vi "Init DAQs.vi"(8 "error in (no error)":errorcluster, 11 "Timing":T1={"Sampling Rate (Hz)"=1000.0, "Samples to Read"=100, "Sampling Mode"=2} {"Sampling Mode" items=["Finite Samples", "Continuous Samples", "Hardware Timed Single Point"]; "Sampling Rate (Hz)" format="%0.2f"}) -> (0 "error out":errorcluster, 2 "Channel Array":refnum<k21>[](array[refnum]))   [LabVIEW 2017]
uses:
  Controls/Timing Controls.ctl
  <vilib>/DAQmx/create/channels.llb/DAQmx Create Channel (AI-Voltage-Basic).vi
  <vilib>/DAQmx/configure/timing.llb/DAQmx Timing (Sample Clock).vi
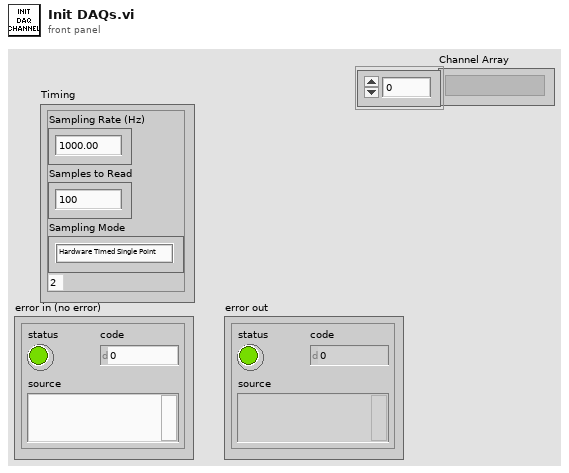
[diagram p1: front panel]
types:
  T1 = typedef "Timing Controls.ctl" = cluster{"Sampling Rate (Hz)":dbl, "Samples to Read":i32, "Sampling Mode":i32}
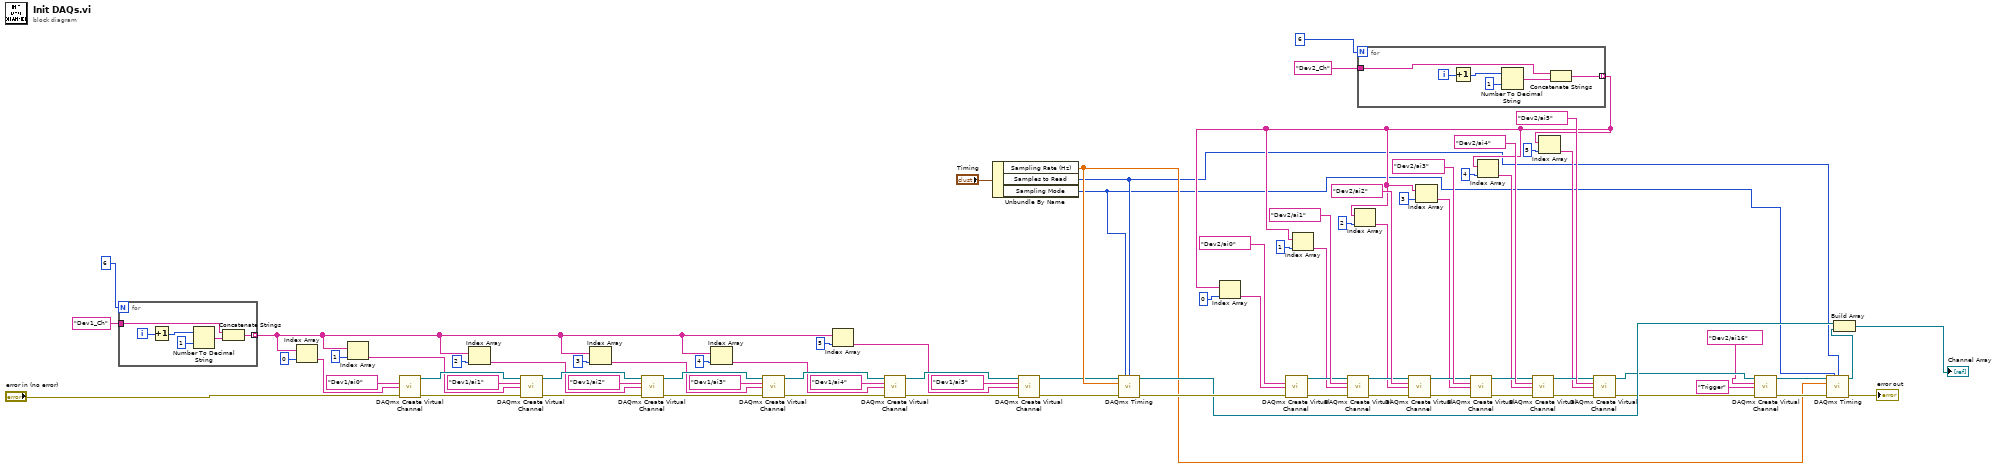
[diagram p0: block diagram]
diagram:
  n1 = for {
    N: 6 -> [_]
    tunnel: "Dev1_Ch" ("name to assign") -> [w82]
    tunnel: [w81] -> w6 mode=indexing
    i -> [w86]
    n2 = Increment(x=w86) -> (x+1=w84:i32)
    n3 = Number To Decimal String(number=w84, width (-)=i16 1) -> (decimal integer string=w83:string)
    n4 = Concatenate Strings(w82, w83) -> (w81:string)
  }
  n5 = Index Array(array=w6, index=0) -> (element=w12:string)
  n6 = Index Array(array=w6, index=1) -> (element=w5:string)
  n7 = call-poly <vilib>:"DAQmx Create Virtual Channel.vi"("physical channels"=tag "Dev1/ai0", "name to assign"=w12, "error in"="error in (no error)") -> ("task out"=w33:refnum<k21>, "error out"=w29:errorcluster)  [unwired: 11 in]
  n8 = Index Array(array=w6, index=2) -> (element=w4:string)
  n9 = call-poly <vilib>:"DAQmx Create Virtual Channel.vi"("task in"=w33, "physical channels"=tag "Dev1/ai1", "name to assign"=w5, "error in"=w29) -> ("task out"=w31:refnum<k21>, "error out"=w27:errorcluster)  [unwired: 10 in]
  n10 = Index Array(array=w6, index=3) -> (element=w3:string)
  n11 = call-poly <vilib>:"DAQmx Create Virtual Channel.vi"("task in"=w31, "physical channels"=tag "Dev1/ai2", "name to assign"=w4, "error in"=w27) -> ("task out"=w30:refnum<k21>, "error out"=w25:errorcluster)  [unwired: 10 in]
  n12 = Index Array(array=w6, index=4) -> (element=w2:string)
  n13 = call-poly <vilib>:"DAQmx Create Virtual Channel.vi"("task in"=w30, "physical channels"=tag "Dev1/ai3", "name to assign"=w3, "error in"=w25) -> ("task out"=w22:refnum<k21>, "error out"=w23:errorcluster)  [unwired: 10 in]
  n14 = Index Array(array=w6, index=5) -> (element=w1:string)
  n15 = call-poly <vilib>:"DAQmx Create Virtual Channel.vi"("task in"=w22, "physical channels"=tag "Dev1/ai4", "name to assign"=w2, "error in"=w23) -> ("task out"=w19:refnum<k21>, "error out"=w18:errorcluster)  [unwired: 10 in]
  n16 = Unbundle By Name("Timing") -> ("Sampling Rate (Hz)"=w37:dbl, "Samples to Read"=w36:i32, "Sampling Mode"=w35:i32)
  n17 = call-poly <vilib>:"DAQmx Create Virtual Channel.vi"("task in"=w19, "physical channels"=tag "Dev1/ai5", "name to assign"=w1, "error in"=w18) -> ("task out"=w17:refnum<k21>, "error out"=w16:errorcluster)  [unwired: 10 in]
  n18 = call-poly <vilib>:"DAQmx Timing.vi"("task/channels in"=w17, "sample mode"=w35, "samples per channel"=w36, "rate"=w37, "error in"=w16) -> ("task out"=w76:refnum<k21>, "error out"=w78:errorcluster)  [unwired: 9 in]
  n19 = for {
    N: 6 -> [_]
    tunnel: "Dev2_Ch" ("name to assign") -> [w88]
    tunnel: [w87] -> w45 mode=indexing
    i -> [w92]
    n20 = Increment(x=w92) -> (x+1=w90:i32)
    n21 = Number To Decimal String(number=w90, width (-)=i16 1) -> (decimal integer string=w89:string)
    n22 = Concatenate Strings(w88, w89) -> (w87:string)
  }
  n23 = Index Array(array=w45, index=0) -> (element=w46:string)
  n24 = call-poly <vilib>:"DAQmx Create Virtual Channel.vi"("physical channels"=tag "Dev2/ai0", "name to assign"=w46, "error in"=w78) -> ("task out"=w61:refnum<k21>, "error out"=w62:errorcluster)  [unwired: 11 in]
  n25 = Index Array(array=w45, index=1) -> (element=w44:string)
  n26 = call-poly <vilib>:"DAQmx Create Virtual Channel.vi"("task in"=w61, "physical channels"=tag "Dev2/ai1", "name to assign"=w44, "error in"=w62) -> ("task out"=w60:refnum<k21>, "error out"=w59:errorcluster)  [unwired: 10 in]
  n27 = Index Array(array=w45, index=2) -> (element=w43:string)
  n28 = call-poly <vilib>:"DAQmx Create Virtual Channel.vi"("task in"=w60, "physical channels"=tag "Dev2/ai2", "name to assign"=w43, "error in"=w59) -> ("task out"=w57:refnum<k21>, "error out"=w58:errorcluster)  [unwired: 10 in]
  n29 = Index Array(array=w45, index=3) -> (element=w42:string)
  n30 = call-poly <vilib>:"DAQmx Create Virtual Channel.vi"("task in"=w57, "physical channels"=tag "Dev2/ai3", "name to assign"=w42, "error in"=w58) -> ("task out"=w55:refnum<k21>, "error out"=w56:errorcluster)  [unwired: 10 in]
  n31 = Index Array(array=w45, index=4) -> (element=w41:string)
  n32 = call-poly <vilib>:"DAQmx Create Virtual Channel.vi"("task in"=w55, "physical channels"=tag "Dev2/ai4", "name to assign"=w41, "error in"=w56) -> ("task out"=w53:refnum<k21>, "error out"=w54:errorcluster)  [unwired: 10 in]
  n33 = Index Array(array=w45, index=5) -> (element=w40:string)
  n34 = call-poly <vilib>:"DAQmx Create Virtual Channel.vi"("task in"=w53, "physical channels"=tag "Dev2/ai5", "name to assign"=w40, "error in"=w54) -> ("task out"=w70:refnum<k21>, "error out"=w71:errorcluster)  [unwired: 10 in]
  n35 = call-poly <vilib>:"DAQmx Create Virtual Channel.vi"("task in"=w70, "physical channels"=tag "Dev2/ai16", "name to assign"="Trigger", "error in"=w71) -> ("task out"=w73:refnum<k21>, "error out"=w74:errorcluster)  [unwired: 10 in]
  n36 = call-poly <vilib>:"DAQmx Timing.vi"("task/channels in"=w73, "sample mode"=w35, "samples per channel"=w36, "rate"=w37, "error in"=w74) -> ("task out"=w39:refnum<k21>, "error out"=→"error out":errorcluster)  [unwired: 9 in]
  n37 = Build Array(w76, w39) -> (→"Channel Array":refnum<k21>[])
